vi "MGCC_comm_main.vi"() -> ()   [LabVIEW 2016]
uses:
  <vilib>/DNP3/DNP3_Master/Operation Mode.ctl
  <vilib>/DNP3/DNP3_Master/Poll Binary Input Variation.ctl
  <vilib>/DNP3/DNP3_Master/Analog Variation.ctl
  <vilib>/DNP3/DNP3_Master/Poll Analog Input Variation.ctl
  <vilib>/DNP3/DNP3_Master/Response Type.ctl
  <vilib>/DNP3/DNP3_Master/Start Stop.ctl
  <vilib>/DNP3/DNP3_Master/Analog Info.ctl
  Finite State Machine/Sub-VIs/MGCC_FntStaMach_gobal.vi
  Global communication.vi
  Global communication output.vi
  DNP3 communication files/MGCC Communication Files/DNP3_Master_Station_MGCC.lvlib
  <vilib>/DNP3/DNP3_Master.lvlib
  MGCC_Global_communication_inputsettings .vi
  <vilib>/ErrorRing/Error Ring.xnode
  <vilib>/Utility/error.llb/Error Cluster From Error Code.vi
panel:
  in  "BESS2 P":dbl
  in  "Gen P":dbl
  in  "BESS1 P":dbl
  in  "PV P":dbl
  in  "Other":bool[](array[boolean])=[FALSE, FALSE, FALSE, FALSE, FALSE, TRUE]
  out "element 2":dbl format="%#_13g"
  out "element":dbl format="%#_15g"
  in  "Gen on off":bool
  out "millisecond timer value":u32
  in  "BESS2 on off":bool
  out "Analog command":T1[][](array[typedef])=[[{"index"=0, "value"=0.0}, {"index"=1, "value"=0.0}, {"index"=2, "value"=0.0}, {"index"=3, "value"=0.0}, {"index"=4, "value"=0.0}, {"index"=5, "value"=0.0}, {"index"=6, "value"=0.0}, {"index"=7, "value"=0.0}, {"index"=0, "value"=0.0}, {"index"=0, "value"=0.0}, {"index"=0, "value"=0.0}, {"index"=0, "value"=0.0}, {"index"=0, "value"=0.0}, {"index"=0, "value"=0.0}, {"index"=0, "value"=0.0}, {"index"=0, "value"=0.0}, {"index"=0, "value"=0.0}, {"index"=0, "value"=0.0}, {"index"=0, "value"=0.0}, {"index"=0, "value"=0.0}, {"index"=0, "value"=0.0}, {"index"=0, "value"=0.0}, {"index"=0, "value"=0.0}, {"index"=0, "value"=0.0}, {"index"=0, "value"=0.0}, {"index"=0, "value"=0.0}, {"index"=0, "value"=0.0}, {"index"=0, "value"=0.0}, {"index"=0, "value"=0.0}, {"index"=0, "value"=0.0}], [{"index"=0, "value"=1.0}, {"index"=1, "value"=0.0}, {"index"=2, "value"=0.0}, {"index"=3, "value"=0.0}, {"index"=4, "value"=0.0}, {"index"=5, "value"=0.0}, {"index"=6, "value"=0.0}, {"index"=7, "value"=0.0}, {"index"=8, "value"=0.0}, {"index"=9, "value"=0.0}, {"index"=10, "value"=1.0}, {"index"=11, "value"=0.0}, {"index"=12, "value"=0.0}, {"index"=13, "value"=0.0}, {"index"=14, "value"=0.0}, {"index"=15, "value"=0.0}, {"index"=16, "value"=0.0}, {"index"=17, "value"=0.0}, {"index"=18, "value"=0.0}, {"index"=19, "value"=0.0}, {"index"=20, "value"=0.0}, {"index"=21, "value"=0.0}, {"index"=22, "value"=0.0}, {"index"=23, "value"=0.0}, {"index"=24, "value"=0.0}, {"index"=25, "value"=0.0}, {"index"=26, "value"=0.0}, {"index"=27, "value"=0.0}, {"index"=28, "value"=0.0}, {"index"=29, "value"=0.0}], [{"index"=0, "value"=1.0}, {"index"=1, "value"=0.0}, {"index"=2, "value"=0.0}, {"index"=3, "value"=0.0}, {"index"=4, "value"=0.0}, {"index"=5, "value"=0.0}, {"index"=6, "value"=0.0}, {"index"=7, "value"=0.0}, {"index"=8, "value"=0.0}, {"index"=9, "value"=0.0}, {"index"=0, "value"=0.0}, {"index"=0, "value"=0.0}, {"index"=0, "value"=0.0}, {"index"=0, "value"=0.0}, {"index"=0, "value"=0.0}, {"index"=0, "value"=0.0}, {"index"=0, "value"=0.0}, {"index"=0, "value"=0.0}, {"index"=0, "value"=0.0}, {"index"=0, "value"=0.0}, {"index"=0, "value"=0.0}, {"index"=0, "value"=0.0}, {"index"=0, "value"=0.0}, {"index"=0, "value"=0.0}, {"index"=0, "value"=0.0}, {"index"=0, "value"=0.0}, {"index"=0, "value"=0.0}, {"index"=0, "value"=0.0}, {"index"=0, "value"=0.0}, {"index"=0, "value"=0.0}]] {"value" format="%#_15f"}
  out "Analog Input 3":dbl[](array[numeric])=[0.0, 0.9942618583829594, 1.0001042537592353, 1.0057560606347744, 0.000339122595439996, 0.0004791410400245842, 0.0008348392532100933, 59.99916524340338, 59.947156617325426, 2.717283070965033, 0.00015278200018709444, -7.123436925011697e-08, 0.0, 0.0, 0.0, 0.0, 0.00033913312014400264, 0.0004791153238902122, 0.0008348307722615329, 4.282069400587955e-07, 4.985840358304346e-07, 1.0429850076204365e-06, 59.94715659629209, 59.94905915422042, -0.15889133301638747, 7.411408048091064e-11, 7.148414556889509e-15, 0.0, 0.0, 0.0, 0.0, 0.00033956781057346825, 0.0004788659040752981, 0.000835003196198178, 1.063294798850192, 0.9804226659808449, 1.0659806618953438, 59.94719306165103, 59.98302369947874, -0.2159221057021128, -8.429146107164405e-08, -1.427083545010438e-08, 0.0, 0.0, 0.0, 0.0, 0.00033909459301970524, 0.0004791936139860199, 0.0008348631578916183, 5.653331029079946e-07, 6.600727141525967e-07, 1.357194267764842e-06, 59.94715897696543, 59.94891873278328, -0.18916293881394353, 7.409342773801824e-11, 1.1504407229014506e-14, 0.0, 0.0, 0.0, 0.0, 0.000339095734403488, 0.0004791957386209789, 0.0008348655488295841, 1.839569633862611e-07, 2.1493942739428542e-07, 4.422781944829691e-07, 59.94715896582638, 59.948980263380776, -0.2257567623665988, 7.41726158569388e-11, 4.555747121595991e-15, 0.0, 0.0, 0.0, 0.0, 1.8399165630995902e-07, 2.1478488850041284e-07, 4.4219588987092504e-07, 6.415774786434966e-11, 6.120015633183977e-11, 1.5017272102437864e-10, 59.948980178541134, 59.95073734635259, -0.13958050074379713, 1.9844258378868394e-17, 4.494075267469924e-22, 0.0, 0.0, 0.0, 0.0, 0.00033884739110626985, 0.00047973946656970325, 0.000835116655298238, 4.794540398320527e-06, 1.6946200635754802, 1.72911748501882, 59.947176698087354, 59.963130270567625, 0.782636575168802, -1.1743140350345762e-07, -6.601684719983745e-08, 0.0, 0.0, 0.0, 0.0, 0.0, 0.0, 0.0, 0.0, 0.0, 0.0, 0.0, 0.0, 0.0, 0.0, 0.0, 0.0, 0.0, 0.0]
  in  "LC1_MS_Network_Settings 3":T2={"Outstation IP"="160.36.56.200", "DNP3 Port"=18000, "DNP3 Master Address"=3, "DNP3 Outstation Address"=1}
  in  "LC1_MS_DNP3_Settings 3":T7={"Binary Out Mode"=6, "Binary In Variation"=0, "Analog Out Variation"=4, "Analog Out Mode"=6, "Analog In Variation"=6} {"Analog In Variation" items=["Default", "32-bit with Flag", "16-bit with Flag", "32-bit without Flag", "16-bit without Flag", "Single-prec with Flag", "Double-prec with Flag"]; "Analog Out Mode" items=["SBO"=0, "Select"=3, "Operate"=4, "Direct"=5, "Direct No Ack"=6]; "Analog Out Variation" items=["32-bit"=1, "16-bit"=2, "Single-prec"=3, "Double-prec"=4]; "Binary In Variation" items=["Default", "Packed Format", "With Flags"]; "Binary Out Mode" items=["SBO"=0, "Select"=3, "Operate"=4, "Direct"=5, "Direct No Ack"=6]}
  in  "ENABLE MS 3":bool=TRUE
  out "LC1_MS_TX_Status_Binary 3":T8=enum."Cancel"
  out "LC1_MS_TX_Status_Analog 3":T8=enum."Success"
  out "LC1_MS_RX_Status_Binary 3":T8=enum."Cancel"
  out "LC1_MS_RX_Status_Analog 3":T8=enum."Success"
  in  "Poll Enable 3":T9={"En_Rx_An"=TRUE, "En_Tx_An"=TRUE, "En_Rx_Di"=FALSE, "En_Tx_Di"=FALSE}
  in  "RESET MS 3":bool caption="Reset Outstation"
  out "Array":T11(array[cluster])=[{"DNP3 channel"="Master/Channel 160.36.56.200: 18000", "DNP3 master"="Master", "DNP3 master session"="Master/Channel 160.36.56.200: 18000/Master Session 3-1", "DNP3 command"="Master/Channel 160.36.56.200: 18000/Master Session 3-1/Command ", "MS_Network_Settings_Initial"={"Outstation IP"="160.36.56.200", "DNP3 Port"=18000, "DNP3 Master Address"=3, "DNP3 Outstation Address"=1}, "Ping status"=enum."Success", "PollD"=[{"start"=0, "stop"=0}], "PollA"=[{"start"=0, "stop"=119}], "error out"={"status"=FALSE, "code"=5103, "source"="DNP3_Master_Station_MGCC.lvlib:LC1_MS_Main.vi:580001<ERR>\nCommunication timeout\n\n\n<b>Complete call chain:</b>\n     DNP3_Master_Station_MGCC.lvlib:LC1_MS_Main.vi:580001\n     MGCC_comm_main.vi"}, "MS_RESET_IND"=FALSE}, {"DNP3 channel"="Master #1/Channel 160.36.58.216: 18000", "DNP3 master"="Master #1", "DNP3 master session"="Master #1/Channel 160.36.58.216: 18000/Master Session 12345-54321", "DNP3 command"="Master #1/Channel 160.36.58.216: 18000/Master Session 12345-54321/Command ", "MS_Network_Settings_Initial"={"Outstation IP"="160.36.58.216", "DNP3 Port"=18000, "DNP3 Master Address"=12345, "DNP3 Outstation Address"=54321}, "Ping status"=enum."Success", "PollD"=[{"start"=0, "stop"=0}], "PollA"=[{"start"=0, "stop"=0}, {"start"=0, "stop"=0}, {"start"=0, "stop"=0}, {"start"=0, "stop"=0}, {"start"=0, "stop"=0}, {"start"=0, "stop"=0}, {"start"=0, "stop"=0}, {"start"=0, "stop"=0}, {"start"=0, "stop"=0}, {"start"=0, "stop"=0}, {"start"=0, "stop"=0}, {"start"=0, "stop"=0}, {"start"=0, "stop"=0}, {"start"=0, "stop"=0}, {"start"=0, "stop"=0}, {"start"=0, "stop"=0}, {"start"=0, "stop"=0}, {"start"=0, "stop"=0}, {"start"=0, "stop"=0}, {"start"=0, "stop"=0}, {"start"=0, "stop"=0}, {"start"=0, "stop"=0}, {"start"=0, "stop"=0}, {"start"=0, "stop"=0}, {"start"=0, "stop"=0}, {"start"=0, "stop"=0}, {"start"=0, "stop"=0}, {"start"=0, "stop"=0}, {"start"=0, "stop"=0}, {"start"=0, "stop"=0}, {"start"=0, "stop"=0}, {"start"=0, "stop"=0}, {"start"=0, "stop"=0}, {"start"=0, "stop"=0}, {"start"=0, "stop"=0}, {"start"=0, "stop"=0}, {"start"=0, "stop"=0}, {"start"=0, "stop"=0}, {"start"=0, "stop"=0}, {"start"=0, "stop"=0}, {"start"=0, "stop"=0}, {"start"=0, "stop"=0}, {"start"=0, "stop"=0}, {"start"=0, "stop"=0}, {"start"=0, "stop"=0}, {"start"=0, "stop"=0}, {"start"=0, "stop"=0}, {"start"=0, "stop"=0}, {"start"=0, "stop"=0}, {"start"=0, "stop"=0}, {"start"=0, "stop"=0}, {"start"=0, "stop"=0}, {"start"=0, "stop"=0}, {"start"=0, "stop"=0}, {"start"=0, "stop"=0}, {"start"=0, "stop"=0}, {"start"=0, "stop"=0}, {"start"=0, "stop"=0}, {"start"=0, "stop"=0}, {"start"=0, "stop"=0}, {"start"=0, "stop"=0}, {"start"=0, "stop"=0}, {"start"=0, "stop"=0}, {"start"=0, "stop"=0}, {"start"=0, "stop"=0}, {"start"=0, "stop"=0}, {"start"=0, "stop"=0}, {"start"=0, "stop"=0}, {"start"=0, "stop"=0}, {"start"=0, "stop"=0}, {"start"=0, "stop"=0}, {"start"=0, "stop"=0}, {"start"=0, "stop"=0}, {"start"=0, "stop"=0}, {"start"=0, "stop"=0}, {"start"=0, "stop"=0}, {"start"=0, "stop"=0}, {"start"=0, "stop"=0}, {"start"=0, "stop"=0}, {"start"=0, "stop"=0}, {"start"=0, "stop"=0}, {"start"=0, "stop"=0}, {"start"=0, "stop"=0}, {"start"=0, "stop"=0}, {"start"=0, "stop"=0}, {"start"=0, "stop"=0}, {"start"=0, "stop"=0}, {"start"=0, "stop"=0}, {"start"=0, "stop"=0}, {"start"=0, "stop"=0}, {"start"=0, "stop"=0}, {"start"=0, "stop"=0}, {"start"=0, "stop"=0}, {"start"=0, "stop"=0}, {"start"=0, "stop"=0}, {"start"=0, "stop"=0}, {"start"=0, "stop"=0}, {"start"=0, "stop"=0}, {"start"=0, "stop"=0}, {"start"=0, "stop"=0}, {"start"=0, "stop"=19}], "error out"={"status"=FALSE, "code"=0, "source"=""}, "MS_RESET_IND"=FALSE}, {"DNP3 channel"="Master #2/Channel 160.36.58.123: 18000", "DNP3 master"="Master #2", "DNP3 master session"="Master #2/Channel 160.36.58.123: 18000/Master Session 12340-54320", "DNP3 command"="Master #2/Channel 160.36.58.123: 18000/Master Session 12340-54320/Command ", "MS_Network_Settings_Initial"={"Outstation IP"="160.36.58.123", "DNP3 Port"=18000, "DNP3 Master Address"=12340, "DNP3 Outstation Address"=54320}, "Ping status"=enum."Success", "PollD"=[{"start"=0, "stop"=0}], "PollA"=[{"start"=0, "stop"=0}, {"start"=0, "stop"=0}, {"start"=0, "stop"=0}, {"start"=0, "stop"=0}, {"start"=0, "stop"=0}, {"start"=0, "stop"=0}, {"start"=0, "stop"=0}, {"start"=0, "stop"=0}, {"start"=0, "stop"=0}, {"start"=0, "stop"=0}, {"start"=0, "stop"=0}, {"start"=0, "stop"=0}, {"start"=0, "stop"=0}, {"start"=0, "stop"=0}, {"start"=0, "stop"=0}, {"start"=0, "stop"=0}, {"start"=0, "stop"=0}, {"start"=0, "stop"=0}, {"start"=0, "stop"=0}, {"start"=0, "stop"=0}, {"start"=0, "stop"=0}, {"start"=0, "stop"=0}, {"start"=0, "stop"=0}, {"start"=0, "stop"=0}, {"start"=0, "stop"=0}, {"start"=0, "stop"=0}, {"start"=0, "stop"=0}, {"start"=0, "stop"=0}, {"start"=0, "stop"=0}, {"start"=0, "stop"=0}, {"start"=0, "stop"=0}, {"start"=0, "stop"=0}, {"start"=0, "stop"=0}, {"start"=0, "stop"=0}, {"start"=0, "stop"=0}, {"start"=0, "stop"=0}, {"start"=0, "stop"=0}, {"start"=0, "stop"=0}, {"start"=0, "stop"=0}, {"start"=0, "stop"=0}, {"start"=0, "stop"=0}, {"start"=0, "stop"=0}, {"start"=0, "stop"=0}, {"start"=0, "stop"=0}, {"start"=0, "stop"=0}, {"start"=0, "stop"=0}, {"start"=0, "stop"=0}, {"start"=0, "stop"=0}, {"start"=0, "stop"=0}, {"start"=0, "stop"=0}, {"start"=0, "stop"=0}, {"start"=0, "stop"=0}, {"start"=0, "stop"=0}, {"start"=0, "stop"=0}, {"start"=0, "stop"=0}, {"start"=0, "stop"=0}, {"start"=0, "stop"=0}, {"start"=0, "stop"=0}, {"start"=0, "stop"=0}, {"start"=0, "stop"=0}, {"start"=0, "stop"=0}, {"start"=0, "stop"=0}, {"start"=0, "stop"=0}, {"start"=0, "stop"=0}, {"start"=0, "stop"=0}, {"start"=0, "stop"=0}, {"start"=0, "stop"=0}, {"start"=0, "stop"=0}, {"start"=0, "stop"=0}, {"start"=0, "stop"=0}, {"start"=0, "stop"=0}, {"start"=0, "stop"=0}, {"start"=0, "stop"=0}, {"start"=0, "stop"=0}, {"start"=0, "stop"=0}, {"start"=0, "stop"=0}, {"start"=0, "stop"=0}, {"start"=0, "stop"=0}, {"start"=0, "stop"=0}, {"start"=0, "stop"=0}, {"start"=0, "stop"=0}, {"start"=0, "stop"=0}, {"start"=0, "stop"=0}, {"start"=0, "stop"=0}, {"start"=0, "stop"=0}, {"start"=0, "stop"=0}, {"start"=0, "stop"=0}, {"start"=0, "stop"=0}, {"start"=0, "stop"=0}, {"start"=0, "stop"=0}, {"start"=0, "stop"=0}, {"start"=0, "stop"=0}, {"start"=0, "stop"=0}, {"start"=0, "stop"=0}, {"start"=0, "stop"=0}, {"start"=0, "stop"=0}, {"start"=0, "stop"=0}, {"start"=0, "stop"=0}, {"start"=0, "stop"=0}, {"start"=0, "stop"=0}, {"start"=0, "stop"=0}, {"start"=0, "stop"=0}, {"start"=0, "stop"=0}, {"start"=0, "stop"=0}, {"start"=0, "stop"=0}, {"start"=0, "stop"=0}, {"start"=0, "stop"=0}, {"start"=0, "stop"=0}, {"start"=0, "stop"=0}, {"start"=0, "stop"=0}, {"start"=0, "stop"=0}, {"start"=0, "stop"=0}, {"start"=0, "stop"=0}, {"start"=0, "stop"=0}, {"start"=0, "stop"=5}], "error out"={"status"=FALSE, "code"=0, "source"=""}, "MS_RESET_IND"=FALSE}]
  out "Active Station":i32=2
  out "error out 3":errorcluster
  out "error out 2":errorcluster
  out "error out":errorcluster
  out "Analog Input 2":dbl[](array[numeric])=[0.0, 1.0369912716646734, 77.34322814800805, 0.0, 0.0, 0.5, 0.0, 0.0, 0.0, 0.0, 0.0, 0.0, 0.0, 0.0, 0.0, 0.0, 0.0, 0.0, 0.0, 0.0, 0.0, 0.0, 0.0, 0.0, 0.0, 0.0, 0.0, 0.0, 0.0, 0.0, 0.0, 0.0, 0.0, 0.0, 0.0, 0.0, 0.0, 0.0, 0.0, 0.0, 0.0, 0.0, 0.0, 0.0, 0.0, 0.0, 0.0, 0.0, 0.0, 0.0, 0.0, 0.0, 0.0, 0.0, 0.0, 0.0, 0.0, 0.0, 0.0, 0.0, 0.0, 0.0, 0.0, 0.0, 0.0, 0.0, 0.0, 0.0, 0.0, 0.0, 0.0, 0.0, 0.0, 0.0, 0.0, 0.0, 0.0, 0.0, 0.0, 0.0, 0.0, 0.0, 0.0, 0.0, 0.0, 0.0, 0.0, 0.0, 0.0, 0.0, 0.0, 0.0, 0.0, 0.0, 0.0, 0.0, 0.0, 0.0, 0.0, 0.0, 0.0, 0.0, 0.0, 0.0, 0.0, 0.0, 0.0, 0.0, 0.0, 0.0, 0.0, 0.0, 0.0, 0.0, 0.0, 0.0, 0.0, 0.0, 0.0, 0.0]
  out "Analog Input":ext[](array[numeric])=[1.0, 0.9417947239708155, 89.67650077398866, -10.0, -1.8175943235401064, 0.5, 0.0, 1.080207045422867, 59.972853370476514, -4.389788955450058e-06, 5.513196811079979e-06, 0.0, 0.0, 0.0, 0.0, 0.0, 0.0, 0.0, 0.0, 0.0, 1.0, 1.0, 1.0, 1.0, 1.0, 1.0, 1.0, 1.0, 1.0, 1.0, 1.0, 1.0, 1.0, 1.0, 1.0, 1.0, 1.0, 1.0, 1.0, 1.0, 1.0, 1.0, 1.0, 1.0, 1.0, 1.0, 1.0, 1.0, 1.0, 1.0, 1.0, 1.0, 1.0, 1.0, 1.0, 1.0, 1.0, 1.0, 1.0, 1.0, 1.0, 1.0, 1.0, 1.0, 1.0, 1.0, 1.0, 1.0, 1.0, 1.0, 1.0, 1.0, 1.0, 1.0, 1.0, 1.0, 1.0, 1.0, 1.0, 1.0, 1.0, 1.0, 1.0, 1.0, 1.0, 1.0, 1.0, 1.0, 1.0, 1.0, 1.0, 1.0, 1.0, 1.0, 1.0, 1.0, 1.0, 1.0, 1.0, 1.0, 1.0, 1.0, 1.0, 1.0, 1.0, 1.0, 1.0, 1.0, 1.0, 1.0, 1.0, 1.0, 1.0, 1.0, 1.0, 1.0, 1.0, 1.0, 1.0, 1.0]
  in  "LC1_MS_Network_Settings 2":T2={"Outstation IP"="10.38.59.112", "DNP3 Port"=18000, "DNP3 Master Address"=12340, "DNP3 Outstation Address"=54320}
  in  "LC1_MS_DNP3_Settings 2":T7={"Binary Out Mode"=6, "Binary In Variation"=0, "Analog Out Variation"=4, "Analog Out Mode"=6, "Analog In Variation"=6} {"Analog In Variation" items=["Default", "32-bit with Flag", "16-bit with Flag", "32-bit without Flag", "16-bit without Flag", "Single-prec with Flag", "Double-prec with Flag"]; "Analog Out Mode" items=["SBO"=0, "Select"=3, "Operate"=4, "Direct"=5, "Direct No Ack"=6]; "Analog Out Variation" items=["32-bit"=1, "16-bit"=2, "Single-prec"=3, "Double-prec"=4]; "Binary In Variation" items=["Default", "Packed Format", "With Flags"]; "Binary Out Mode" items=["SBO"=0, "Select"=3, "Operate"=4, "Direct"=5, "Direct No Ack"=6]}
  in  "ENABLE MS 2":bool=TRUE
  out "MS SETTINGS CHANGED 2":bool
  out "LC1_MS_TX_Status_Binary 2":T8=enum."Cancel"
  out "LC1_MS_TX_Status_Analog 2":T8=enum."Success"
  out "LC1_MS_RX_Status_Binary 2":T8=enum."Cancel"
  out "LC1_MS_RX_Status_Analog 2":T8=enum."Success"
  out "RESET MS IND 2":bool
  in  "Poll Enable 2":T9={"En_Rx_An"=TRUE, "En_Tx_An"=TRUE, "En_Rx_Di"=FALSE, "En_Tx_Di"=FALSE}
  in  "RESET MS 2":bool caption="Reset Outstation"
  in  "Poll Enable":T9={"En_Rx_An"=TRUE, "En_Tx_An"=TRUE, "En_Rx_Di"=FALSE, "En_Tx_Di"=FALSE}
  out "Numeric":i32=132
  out "RESET MS IND":bool
  out "LC1_MS_RX_Status_Analog":T8=enum."Success"
  out "LC1_MS_RX_Status_Binary":T8=enum."Cancel"
  out "LC1_MS_TX_Status_Analog":T8=enum."Success"
  out "LC1_MS_TX_Status_Binary":T8=enum."Cancel"
  out "MS SETTINGS CHANGED":bool
  in  "RESET MS":bool caption="Reset Outstation"
  in  "ENABLE MS":bool=TRUE
  in  "LC1_MS_DNP3_Settings":T7={"Binary Out Mode"=6, "Binary In Variation"=0, "Analog Out Variation"=4, "Analog Out Mode"=6, "Analog In Variation"=6} {"Analog In Variation" items=["Default", "32-bit with Flag", "16-bit with Flag", "32-bit without Flag", "16-bit without Flag", "Single-prec with Flag", "Double-prec with Flag"]; "Analog Out Mode" items=["SBO"=0, "Select"=3, "Operate"=4, "Direct"=5, "Direct No Ack"=6]; "Analog Out Variation" items=["32-bit"=1, "16-bit"=2, "Single-prec"=3, "Double-prec"=4]; "Binary In Variation" items=["Default", "Packed Format", "With Flags"]; "Binary Out Mode" items=["SBO"=0, "Select"=3, "Operate"=4, "Direct"=5, "Direct No Ack"=6]}
  in  "LC1_MS_Network_Settings":T2={"Outstation IP"="10.38.59.111", "DNP3 Port"=18000, "DNP3 Master Address"=12345, "DNP3 Outstation Address"=54321}
  in  "Manually control Relays":bool
  in  "PV on off":bool
  in  "Manually control sources":bool
  in  "BESS1 on off":bool
  in  "Relay":bool[](array[boolean])=[FALSE, FALSE, FALSE, FALSE, FALSE, FALSE, FALSE, FALSE, FALSE, FALSE]
  # "Copyright <2020> <The University of Tennessee at Knoxville and the University of Tennessee Research Foundation>\n\nRedistribution and use in source and binary forms, with or without modification, are permitted provided that the following conditions are met:\n\n1. Redistributions of source code must retain the above copyright notice, this list of conditions and the following disclaimer.\n\n2. Redistributions in binary form must reproduce the above copyright notice, this list of conditions and the following disclaimer in the documentation and/or other materials provided with the distribution.\n\n3. Neither the name of the copyright holder nor the names of its contributors may be used to endorse or promote products derived from this software without specific prior written permission.\n\nTHIS SOFTWARE IS PROVIDED BY THE COPYRIGHT HOLDERS AND CONTRIBUTORS \"AS IS\" AND ANY EXPRESS OR IMPLIED WARRANTIES, INCLUDING, BUT NOT LIMITED TO, THE IMPLIED WARRANTIES OF MERCHANTABILITY AND FITNESS FOR A PARTICULAR PURPOSE ARE DISCLAIMED. IN NO EVENT SHALL THE COPYRIGHT HOLDER OR CONTRIBUTORS BE LIABLE FOR ANY DIRECT, INDIRECT, INCIDENTAL, SPECIAL, EXEMPLARY, OR CONSEQUENTIAL DAMAGES (INCLUDING, BUT NOT LIMITED TO, PROCUREMENT OF SUBSTITUTE GOODS OR SERVICES; LOSS OF USE, DATA, OR PROFITS; OR BUSINESS INTERRUPTION) HOWEVER CAUSED AND ON ANY THEORY OF LIABILITY, WHETHER IN CONTRACT, STRICT LIABILITY, OR TORT (INCLUDING NEGLIGENCE OR OTHERWISE) ARISING IN ANY WAY OUT OF THE USE OF THIS SOFTWARE, EVEN IF ADVISED OF THE POSSIBILITY OF SUCH DAMAGE."
  # "LC2"
  # "LC1"
  # "IntelliRupter"
  # "Settings Changed; Reset to Update"
  # "1"
  # "fault 3 (L6)"
  # "2"
  # "fault 5 (10)"
  # "3"
  # "fault 6 (L11)"
  # "4"
  # "fault 7 (L8)"
  # "5"
  # "reset"
  # "6"
  # "grid enable"
  # "7"
  # "8"
  # "Gnd trans1"
  # "Gnd trans2"
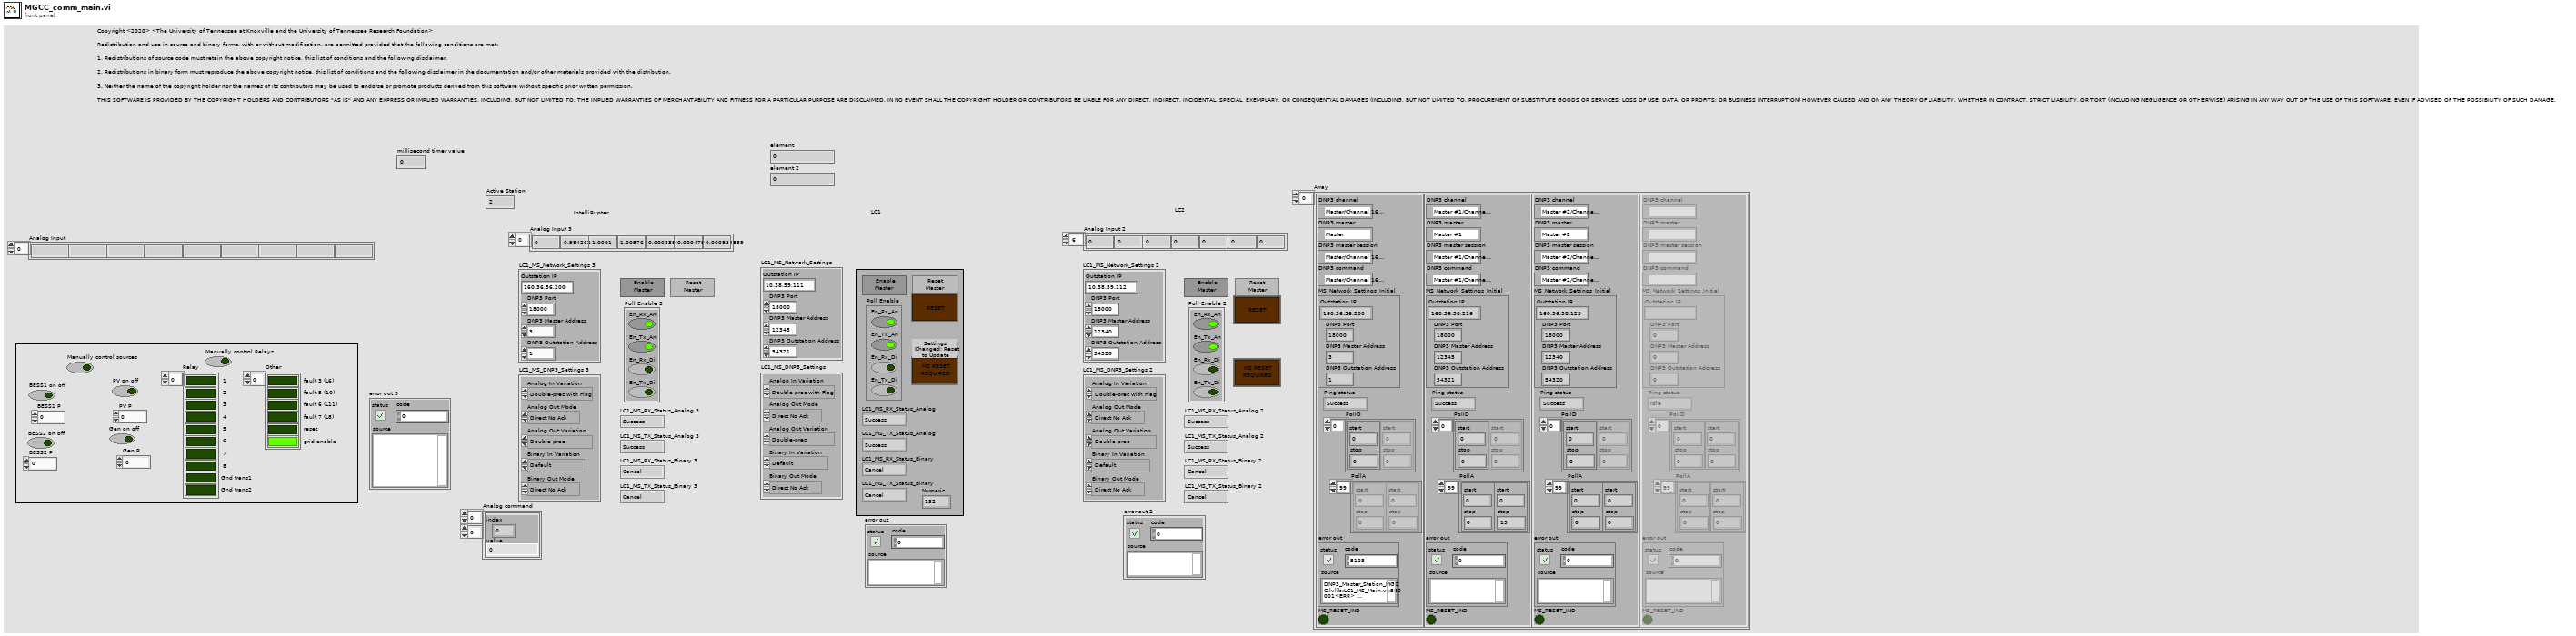
[diagram p1: front panel]
types:
  T1 = typedef "DNP3_Master.lvlib/Analog Info.ctl" = cluster{"index":u16, "value":dbl}
  T2 = cluster{"Outstation IP":string, "DNP3 Port":u16, "DNP3 Master Address":u16, "DNP3 Outstation Address":u16}
  T3 = typedef "DNP3_Master.lvlib/Operation Mode.ctl" = u8
  T4 = typedef "DNP3_Master.lvlib/Poll Binary Input Variation.ctl" = u8
  T5 = typedef "DNP3_Master.lvlib/Analog Variation.ctl" = u8
  T6 = typedef "DNP3_Master.lvlib/Poll Analog Input Variation.ctl" = u8
  T7 = cluster{"Binary Out Mode":T3, "Binary In Variation":T4, "Analog Out Variation":T5, "Analog Out Mode":T3, "Analog In Variation":T6}
  T8 = typedef "DNP3_Master.lvlib/Response Type.ctl" = enum16{"Idle", "Buffering", "Pending", "Success", "Failure", "Mismatch", "Status Code", "IIN", "Timeout", "Cancel"}
  T9 = cluster{"En_Rx_An":bool, "En_Tx_An":bool, "En_Rx_Di":bool, "En_Tx_Di":bool}
  T10 = typedef "DNP3_Master.lvlib/Start Stop.ctl" = cluster{"start":u16, "stop":u16}
  T11 = cluster{"DNP3 channel":refnum<k21>, "DNP3 master":refnum<k21>, "DNP3 master session":refnum<k21>, "DNP3 command":refnum<k21>, "MS_Network_Settings_Initial":cluster{"Outstation IP":string, "DNP3 Port":u16, "DNP3 Master Address":u16, "DNP3 Outstation Address":u16}, "Ping status":T8, "PollD":T10[], "PollA":T10[], "error out":errorcluster, "MS_RESET_IND":bool}[]
  T12 = cluster{"Binary Out Mode":T3, "Binary In Variation":T4, "Analog Out Variation":T5, "Analog Out Mode":T3, "Analog In Variation":T6}[]
  T13 = cluster{"Outstation IP":string, "DNP3 Port":u16, "DNP3 Master Address":u16, "DNP3 Outstation Address":u16}[]
  T14 = cluster{"En_Rx_An":bool, "En_Tx_An":bool, "En_Rx_Di":bool, "En_Tx_Di":bool}[]
  T15 = cluster{"response status":T8, "response status":T8, "response status":T8, "response status":T8}
  T16 = cluster{"DNP3 channel":refnum<k21>, "DNP3 master":refnum<k21>, "DNP3 master session":refnum<k21>, "DNP3 command":refnum<k21>, "MS_Network_Settings_Initial":cluster{"Outstation IP":string, "DNP3 Port":u16, "DNP3 Master Address":u16, "DNP3 Outstation Address":u16}, "Ping status":T8, "PollD":T10[], "PollA":T10[], "error out":errorcluster, "MS_RESET_IND":bool}
  T17 = cluster{string, "DNP3 port BESS":dbl, "DNP3 Master Address BESS":dbl, "DNP3 Outstation Address BESS":dbl}
  T18 = cluster{string, "DNP3 port PV":dbl, "DNP3 Master Address PV":dbl, "DNP3 Outstation Address PV":dbl}
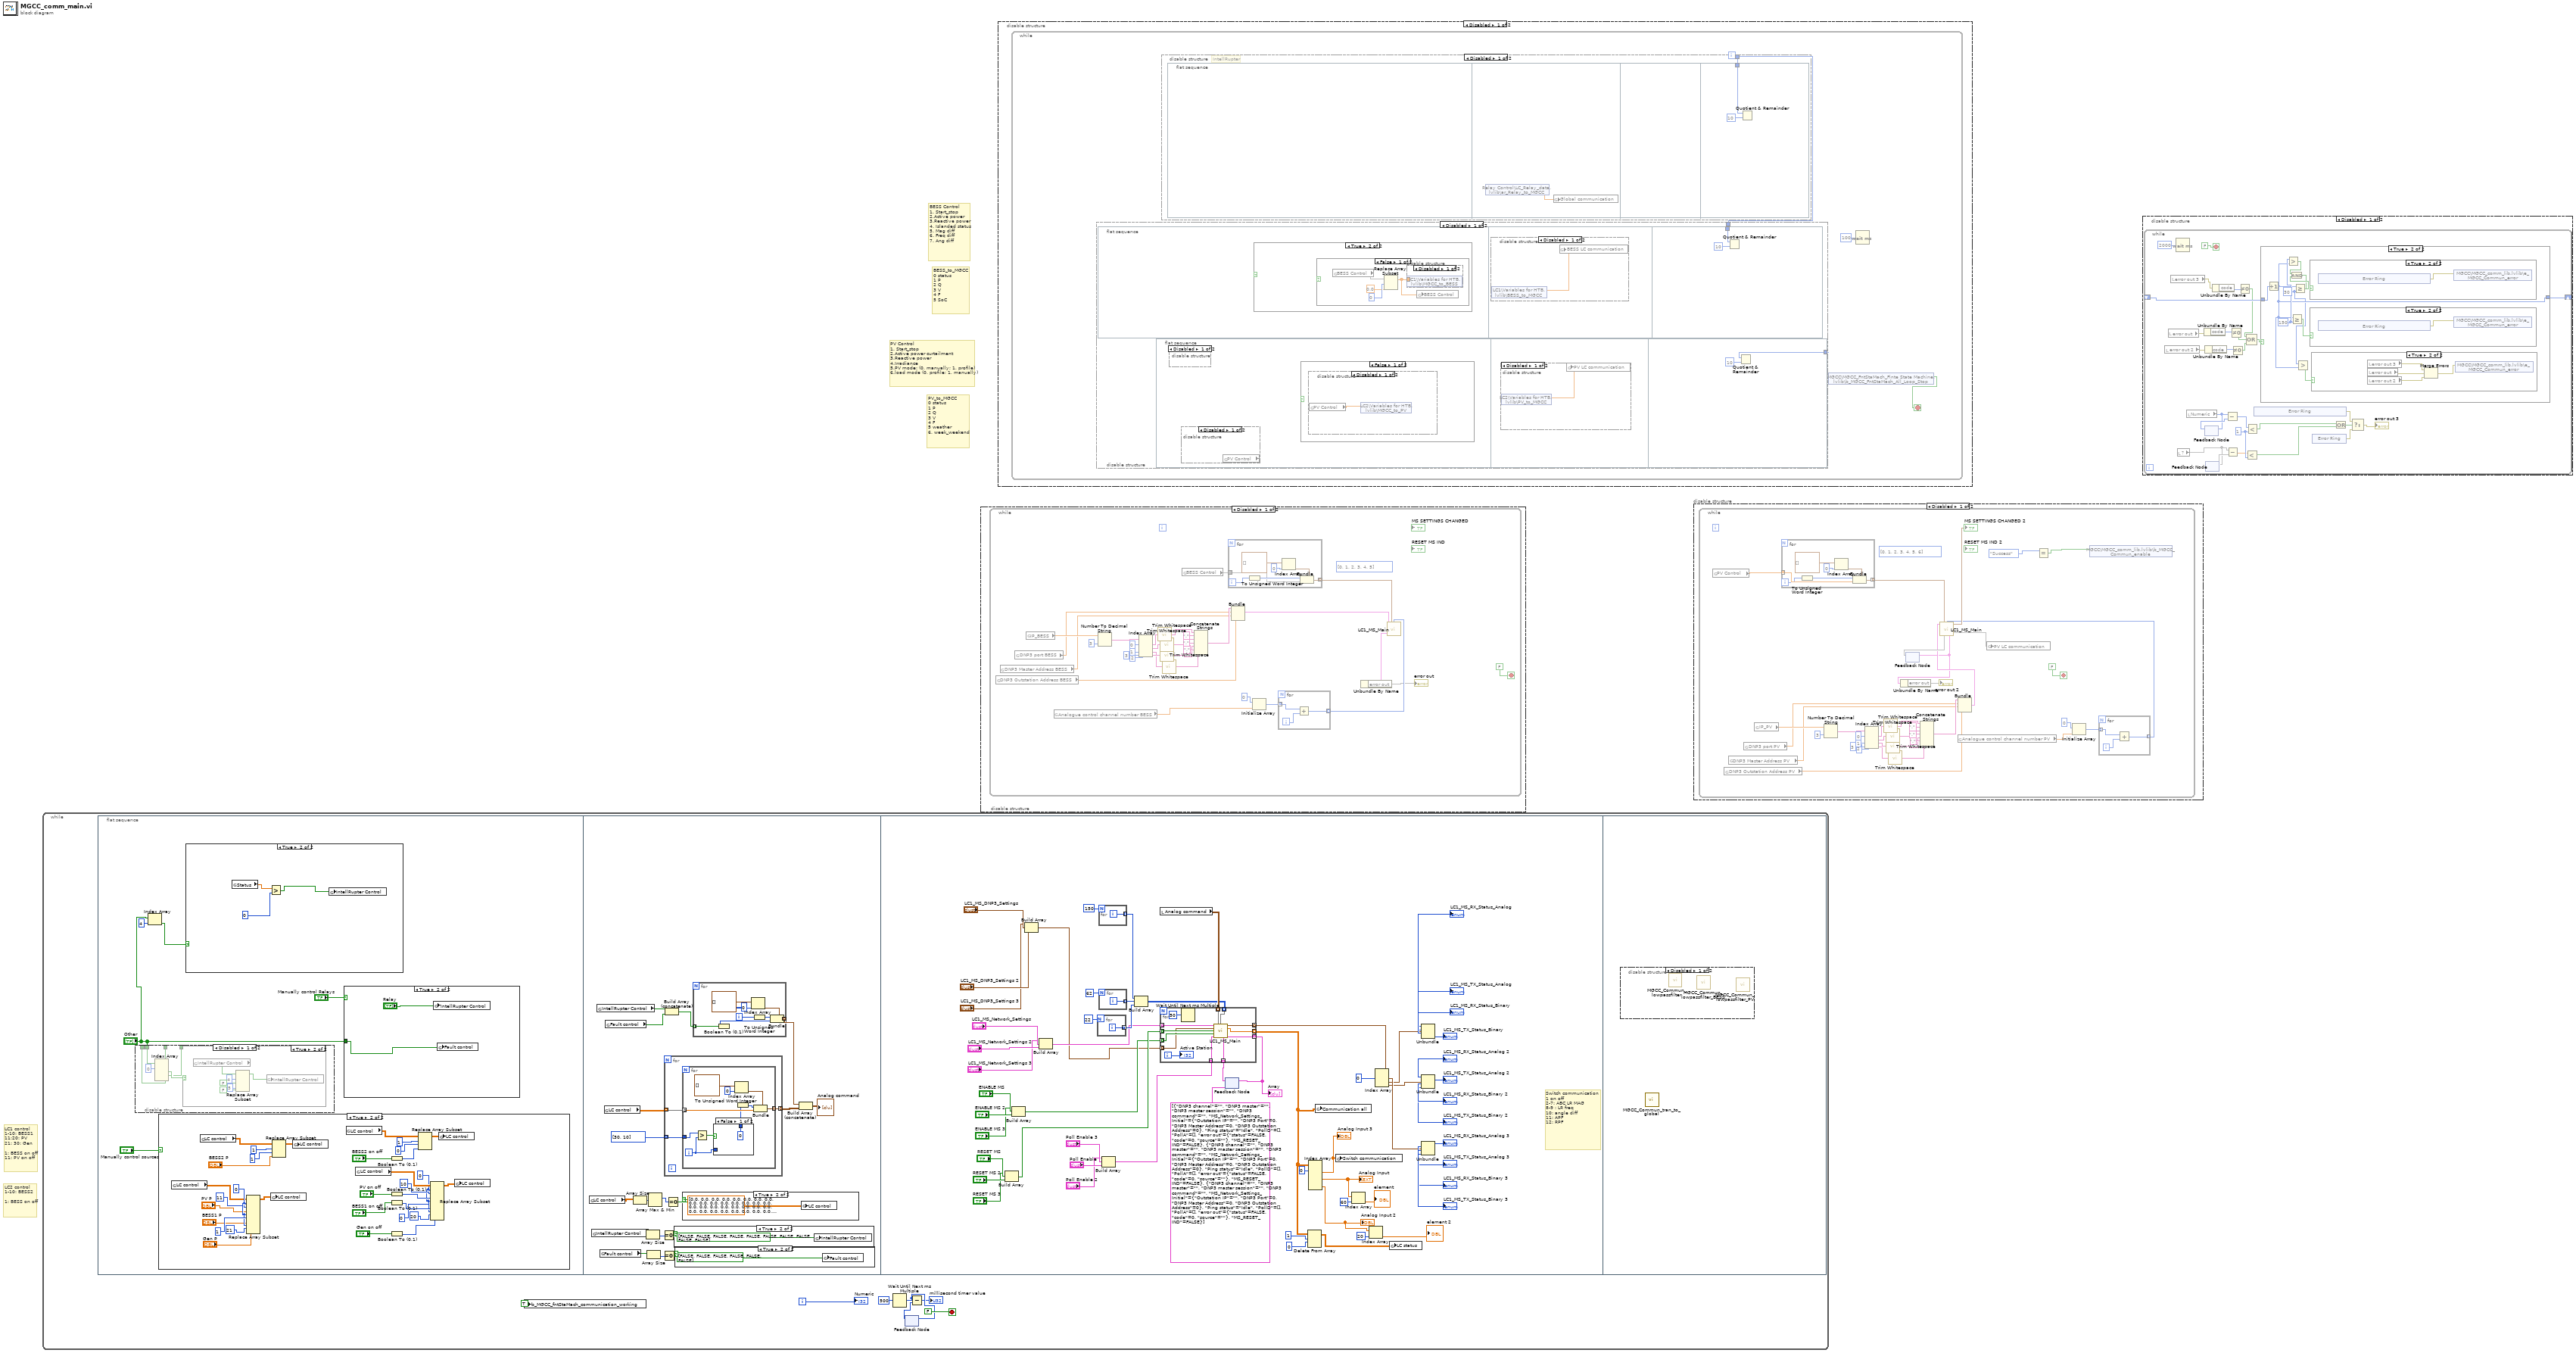
[diagram p0: block diagram]
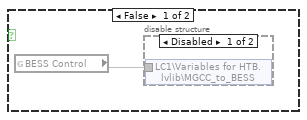
[diagram p2: hidden frame]
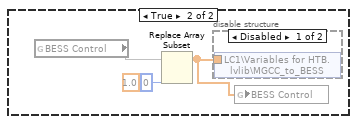
[diagram p5: hidden frame]
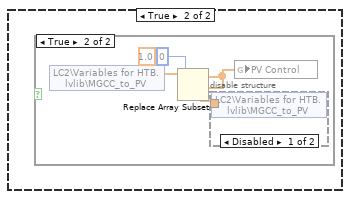
[diagram p9: hidden frame]
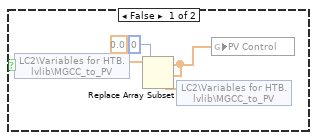
[diagram p10: hidden frame]
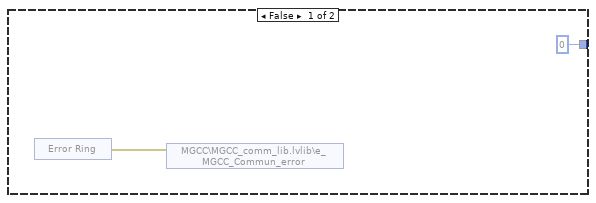
[diagram p18: hidden frame]
diagram:
  # "LC2 control\n1-10: BESS2\n\n1: BESS on off"
  # "LC1 control\n1-10: BESS1\n11:20: PV\n21: 30: Gen\n\n1: BESS on off\n11: PV on off"
  # "PV_to_MGCC\n0 status\n1 P\n2 Q\n3 V\n4 F\n5 weather\n6. week_weekend"
  # "BESS_to_MGCC\n0 status\n1 P\n2 Q\n3 V\n4 F\n5 SoC"
  # "PV Control\n1. Start_stop\n2.Active power curtailment\n3.Reactive power\n4.Irradiance\n5.PV mode: (0, manually; 1, profile)\n6.load mode (0, profile; 1, manually)"
  # "BESS Control\n1. Start_stop\n2.Active power\n3.Reactive power\n4. Islanded status\n5. Mag diff\n6. Freq diff\n7. Ang diff"
  n1 = while {
    i -> [w7]
    stop <- FALSE stop-if-true
    n2 = flat-sequence {
      frame #0 {
        n3 = disable-structure shown="Disabled" {
          disable-tunnel: "Other" -> [w20 _]
          disable-tunnel: [w18 _] -> _
          disable-tunnel: [w17 _] -> _
          disable-tunnel: [w16 _] -> _
          frame Disabled {
            n4 = Index Array(array=w20, index #1=0 ("index")) -> (element #1=w16:bool, element #2=w19:bool, element #3=w18:bool, element #4=w17:bool)  [unwired: 3 in]
            n5 = case shown="True" w19 {
              frame False {
              }
              frame True {
                n6 = global read "Global communication output.vi" "IntellRupter Control"() -> (w27:bool[])
                n7 = Replace Array Subset(array=w27, new element #1=FALSE ("new element/subarray"), index #1=4 ("index"), new element #2=FALSE ("new element/subarray"), index #2=5 ("index")) -> (w26:bool[])
                n8 = global write "Global communication output.vi" "IntellRupter Control"(w26) -> ()
              }
            }
          }
          frame Enabled {
          }
        }
        n9 = Index Array(array="Other", index=4) -> (element=w8:bool)
        n10 = case shown="True" "Manually control sources" {
          frame False {
          }
          frame True {
            w44 = 0 ("index")
            w49 = 0 ("index")
            n11 = global read "Global communication.vi" "LC control"() -> (w41:dbl[][])
            n12 = global read "Global communication.vi" "LC control"() -> (w35:dbl[][])
            n13 = Replace Array Subset(array=w41, new element #1="PV P", index (row) #1=w44, index (col) #1=11 ("index"), new element #2="BESS1 P", index (row) #2=w44, index (col) #2=1 ("index"), new element #3="Gen P", index (row) #3=w44, index (col) #3=21 ("index")) -> (w42:dbl[][])
            n14 = global write "Global communication.vi" "LC control"(w42) -> ()
            n15 = Replace Array Subset(array=w35, new element="BESS2 P", index (row)=1 ("index"), index (col)=1 ("index")) -> (w33:dbl[][])
            n16 = global write "Global communication.vi" "LC control"(w33) -> ()
            n17 = global read "Global communication.vi" "LC control"() -> (w55:dbl[][])
            n18 = global read "Global communication.vi" "LC control"() -> (w53:dbl[][])
            n19 = Boolean To (0,1)(Boolean="BESS2 on off") -> (0, 1=w59:i16)
            n20 = Boolean To (0,1)(Boolean="PV on off") -> (0, 1=w63:i16)
            n21 = Boolean To (0,1)(Boolean="BESS1 on off") -> (0, 1=w57:i16)
            n22 = Boolean To (0,1)(Boolean="Gen on off") -> (0, 1=w56:i16)
            n23 = Replace Array Subset(array=w55, new element=w59, index (row)=1 ("index"), index (col)=0 ("index")) -> (w54:dbl[][])
            n24 = Replace Array Subset(array=w53, new element #1=w63, index (row) #1=w49, index (col) #1=10 ("index"), new element #2=w57, index (row) #2=w49, index (col) #2=0 ("index"), new element #3=w56, index (row) #3=w49, index (col) #3=20 ("index")) -> (w52:dbl[][])
            n25 = global write "Global communication.vi" "LC control"(w54) -> ()
            n26 = global write "Global communication.vi" "LC control"(w52) -> ()
          }
        }
        n27 = case shown="True" w8 {
          frame False {
          }
          frame True {
            n28 = global read "Global communication.vi" "Status"() -> (w15:dbl[])
            n29 = Greater?(x=w15, y=0 ("index")) -> (0:w13:bool[])
            n30 = global write "Global communication output.vi" "IntellRupter Control"(w13) -> ()
          }
        }
        n31 = case shown="True" "Manually control Relays" {
          tunnel: "Other" -> [w28 w31]
          frame False {
            n32 = global read "Global communication output.vi" "IntellRupter Control"() -> (w29:bool[])
            n33 = disable-structure shown="Disabled" {
              frame Disabled {
                n34 = global read "Global communication output.vi" "Fault control"() -> (w30:bool[])
                n35 = local write "Other"(w30) -> ()
              }
              frame Enabled {
              }
            }
            n36 = global write "Global communication output.vi" "Fault control"(w28) -> ()
            n37 = local write "Relay"(w29) -> ()
          }
          frame True {
            n38 = global write "Global communication output.vi" "IntellRupter Control"("Relay") -> ()
            n39 = global write "Global communication output.vi" "Fault control"(w31) -> ()
          }
        }
      }
      frame #1 {
        n40 = global read "Global communication.vi" "LC control"() -> (w75:dbl[][])
        n41 = global read "Global communication output.vi" "IntellRupter Control"() -> (w78:bool[])
        n42 = global read "Global communication output.vi" "IntellRupter Control"() -> (w69:bool[])
        n43 = global read "Global communication output.vi" "Fault control"() -> (w65:bool[])
        n44 = global read "Global communication.vi" "LC control"() -> (w72:dbl[][])
        n45 = global read "Global communication output.vi" "Fault control"() -> (w68:bool[])
        n46 = Array Size(array=w75) -> (size(s)=w74:i32[])
        n47 = Array Size(array=w78) -> (size(s)=w77:i32)
        n48 = Array Size(array=w65) -> (size(s)=w66:i32)
        n49 = Array Max & Min(array=w74) -> (max index (indices)=w73:i32)  [unwired: 3 out]
        n50 = Equal To 0?(x=w77) -> (x = 0?=w76:bool)
        n51 = Equal To 0?(x=w66) -> (x = 0?=w67:bool)
        n52 = for {
          tunnel: [w86] -> w82 mode=indexing
          tunnel: w72 -> [w85] mode=indexing
          tunnel: i32[] [30, 10] ("IntellRupter Control") -> [w84] mode=indexing
          n53 = for {
            tunnel: [w96] -> w86 mode=indexing
            tunnel: w85 -> [w91] mode=indexing
            tunnel: w84 -> [w90]
            i -> [w88]
            n54 = Greater?(x=w90, y=w88) -> (0:w89:bool)
            n55 = case shown="False" w89 {
              tunnel: w88 -> [_ w98]
              tunnel: [0 w98] -> w87
              frame False {
              }
              frame True {
              }
            }
            n56 = Index Array(array=T1[] [] ("values"), index=0) -> (element=w93:T1)
            n57 = To Unsigned Word Integer(number=w87) -> (unsigned 16bit integer=w92:u16)
            n58 = Bundle(cluster=w93, "index"=w92, "value"=w91) -> (w96:T1)
          }
        }
        n59 = Build Array (concatenate)(w69, w68) -> (w70:bool[])
        n60 = Equal To 0?(x=w73) -> (x = 0?=w79:bool)
        n61 = case shown="True" w76 {
          frame False {
          }
          frame True {
            n62 = global write "Global communication output.vi" "IntellRupter Control"(bool[] [FALSE, FALSE, FALSE, FALSE, FALSE, FALSE, FALSE, FALSE, FALSE, FALSE] ("IntellRupter Control")) -> ()
          }
        }
        n63 = case shown="True" w67 {
          frame False {
          }
          frame True {
            n64 = global write "Global communication output.vi" "Fault control"(bool[] [FALSE, FALSE, FALSE, FALSE, FALSE, FALSE] ("IntellRupter Control")) -> ()
          }
        }
        n65 = case shown="True" w79 {
          frame False {
          }
          frame True {
            n66 = global write "Global communication.vi" "LC control"(dbl[][] [[0.0, 0.0, 0.0, 0.0, 0.0, 0.0, 0.0, 0.0, 0.0, 0.0, 0.0, 0.0, 0.0, 0.0, 0.0, 0.0, 0.0, 0.0, 0.0, 0.0, 0.0, 0.0, 0.0, 0.0, 0.0, 0.0, 0.0, 0.0, 0.0, 0.0, 0.0, 0.0, 0.0, 0.0, 0.0, 0.0, 0.0], [0.0, 0.0, 0.0, 0.0, 0.0, 0.0, 0.0, 0.0, 0.0, 0.0, 0.0, 0.0, 0.0, 0.0, 0.0, 0.0, 0.0, 0.0, 0.0, 0.0, 0.0, 0.0, 0.0, 0.0, 0.0, 0.0, 0.0, 0.0, 0.0, 0.0, 0.0, 0.0, 0.0, 0.0, 0.0, 0.0, 0.0]] ("LC control")) -> ()
          }
        }
        n67 = for {
          tunnel: [w108] -> w80 mode=indexing
          tunnel: w70 -> [w101] mode=indexing
          i -> [w103]
          n68 = Boolean To (0,1)(Boolean=w101) -> (0, 1=w102:i16)
          n69 = Index Array(array=T1[] [] ("values"), index=0) -> (element=w105:T1)
          n70 = To Unsigned Word Integer(number=w103) -> (unsigned 16bit integer=w104:u16)
          n71 = Bundle(cluster=w105, "index"=w104, "value"=w102) -> (w108:T1)
        }
        n72 = Build Array (concatenate)(w80, w82) -> (→"Analog command":T1[][])
      }
      frame #2 {
        # "Switch communication\n1 on off\n2-7: ABC LR MAG\n8-9 : LR freq\n10: angle diff\n11: APF\n12: RPF"
        n73 = Build Array("RESET MS 3", "RESET MS", "RESET MS 2") -> (w126:bool[])
        n74 = Build Array("ENABLE MS 3", "ENABLE MS", "ENABLE MS 2") -> (w125:bool[])
        n75 = Build Array("LC1_MS_DNP3_Settings 3", "LC1_MS_DNP3_Settings", "LC1_MS_DNP3_Settings 2") -> (w123:T12)
        n76 = Build Array("LC1_MS_Network_Settings 3", "LC1_MS_Network_Settings", "LC1_MS_Network_Settings 2") -> (w124:T13)
        n77 = for {
          N: 22 -> [_]
          tunnel: [w169] -> w148 mode=indexing
          i -> [w169]
        }
        n78 = for {
          N: 150 -> [_]
          tunnel: [w171] -> w143 mode=indexing
          i -> [w171]
        }
        n79 = for {
          N: 62 -> [_]
          tunnel: [w170] -> w146 mode=indexing
          i -> [w170]
        }
        n80 = Build Array("Poll Enable 2", "Poll Enable 3", "Poll Enable") -> (w127:T14)
        n81 = Build Array(w143, w146, w148) -> (w128:i32[][])
        n82 = local read "Analog command"() -> (w129:T1[][])
        n83 = feedback #1(T11 [{"DNP3 channel"="", "DNP3 master"="", "DNP3 master session"="", "DNP3 command"="", "MS_Network_Settings_Initial"={"Outstation IP"="", "DNP3 Port"=0, "DNP3 Master Address"=0, "DNP3 Outstation Address"=0}, "Ping status"=enum."Idle", "PollD"=[], "PollA"=[], "error out"={"status"=FALSE, "code"=0, "source"=""}, "MS_RESET_IND"=FALSE}, {"DNP3 channel"="", "DNP3 master"="", "DNP3 master session"="", "DNP3 command"="", "MS_Network_Settings_Initial"={"Outstation IP"="", "DNP3 Port"=0, "DNP3 Master Address"=0, "DNP3 Outstation Address"=0}, "Ping status"=enum."Idle", "PollD"=[], "PollA"=[], "error out"={"status"=FALSE, "code"=0, "source"=""}, "MS_RESET_IND"=FALSE}, {"DNP3 channel"="", "DNP3 master"="", "DNP3 master session"="", "DNP3 command"="", "MS_Network_Settings_Initial"={"Outstation IP"="", "DNP3 Port"=0, "DNP3 Master Address"=0, "DNP3 Outstation Address"=0}, "Ping status"=enum."Idle", "PollD"=[], "PollA"=[], "error out"={"status"=FALSE, "code"=0, "source"=""}, "MS_RESET_IND"=FALSE}]) -> (w131:T11)
        n84 = for {
          tunnel: [w184] -> w130 mode=indexing
          tunnel: w131 -> [w179] mode=indexing
          tunnel: [w181] -> w132 mode=indexing
          tunnel: [w180] -> w109 mode=indexing
          tunnel: w129 -> [w178] mode=indexing
          tunnel: w128 -> [w177] mode=indexing
          tunnel: w127 -> [w176] mode=indexing
          tunnel: w126 -> [w175] mode=indexing
          tunnel: w125 -> [w174] mode=indexing
          tunnel: w124 -> [w173] mode=indexing
          tunnel: w123 -> [w172] mode=indexing
          i -> [w183]
          n85 = Wait Until Next ms Multiple(millisecond multiple=u32 50) -> ()  [unwired: 1 out]
          n86 = call "LC1_MS_Main.vi"("MS_Network_Settings"=w173, "Analog Output"=w178, "Analog Input Indexes"=w177, "MS_DNP3_Settings"=w172, "MS_RESET"=w175, "MS_ENABLE"=w174, "Poll Enable"=w176, "DNP3 Session Feedback"=w179) -> ("Comm Status"=w181:T15, "Analog Input"=w180:dbl[], "DNP3 Session Output"=w184:T16)  [unwired: 4 in, 1 out]
          "Active Station" <- w183
        }
        "Array" <- w130
        n87 = feedback-in #1(w130) -> ()
        n88 = Delete From Array(array=w109, length=1 ("index"), index (row)=0 ("index")) -> (array with subset deleted=w116:dbl[][])  [unwired: 1 in, 1 out]
        n89 = Index Array(array=w109, index (row) #1=0 ("index")) -> (element #1=w119:dbl[], element #2=w115:dbl[], element #3=w111:dbl[])  [unwired: 5 in]
        "Analog Input" <- w115
        "Analog Input 2" <- w111
        "Analog Input 3" <- w119
        n90 = global write "Global communication.vi" "Communication all"(w109) -> ()
        n91 = global write "Global communication.vi" "Switch communication"(w119) -> ()
        n92 = Index Array(array=w115, index=60) -> (element=→"element":dbl)
        n93 = Index Array(array=w111, index=20) -> (element=→"element 2":dbl)
        n94 = Index Array(array=w132, index #1=0 ("index")) -> (element #1=w122:T15, element #2=w121:T15, element #3=w120:T15)  [unwired: 2 in]
        n95 = global write "Global communication.vi" "LC status"(w116) -> ()
        n96 = Unbundle(w121) -> ("response status"=→"LC1_MS_RX_Status_Analog":T8, "response status"=→"LC1_MS_TX_Status_Analog":T8, "response status"=→"LC1_MS_RX_Status_Binary":T8, "response status"=→"LC1_MS_TX_Status_Binary":T8)
        n97 = Unbundle(w120) -> ("response status"=→"LC1_MS_RX_Status_Analog 2":T8, "response status"=→"LC1_MS_TX_Status_Analog 2":T8, "response status"=→"LC1_MS_RX_Status_Binary 2":T8, "response status"=→"LC1_MS_TX_Status_Binary 2":T8)
        n98 = Unbundle(w122) -> ("response status"=→"LC1_MS_RX_Status_Analog 3":T8, "response status"=→"LC1_MS_TX_Status_Analog 3":T8, "response status"=→"LC1_MS_RX_Status_Binary 3":T8, "response status"=→"LC1_MS_TX_Status_Binary 3":T8)
      }
      frame #3 {
        n99 = disable-structure shown="Disabled" {
          frame Disabled {
            n100 = call "MGCC_Commun_lowpassfilter.vi"() -> ()  [unwired: 12 in]
            n101 = call "MGCC_Commun_lowpassfilter_BESS.vi"() -> ()  [unwired: 12 in]
            n102 = call "MGCC_Commun_lowpassfilter_PV.vi"() -> ()  [unwired: 12 in]
          }
          frame Enabled {
          }
        }
        n103 = call "MGCC_Commun_tran_to_global.vi"() -> ()  [unwired: 12 in]
      }
    }
    n104 = global write "MGCC_FntStaMach_gobal.vi" "b_MGCC_fntStaMach_communication_working"(TRUE ("b_MGCC_fntStaMach_ModelMgmt_done")) -> ()
    n105 = Wait Until Next ms Multiple(millisecond multiple=u32 500) -> (millisecond timer value=w3:u32)
    n106 = feedback-in #2(w3) -> ()
    n107 = feedback #2() -> (w4:u32)  [unwired: 1 in]
    n108 = Subtract(x=w3, y=w4) -> (x-y=→"millisecond timer value":u32)
    "Numeric" <- w7
  }
  n109 = disable-structure shown="Disabled" {
    frame Disabled {
      n110 = while {
        i -> [w223]
        stop <- FALSE stop-if-true
        (unwired) u16[] [0, 1, 2, 3, 4, 5] ("Analog Input Indexes")
        n111 = global read "MGCC_Global_communication_inputsettings .vi" "DNP3 Outstation Address BESS"() -> (w193:dbl)
        n112 = global read "MGCC_Global_communication_inputsettings .vi" "DNP3 Master Address BESS"() -> (w194:dbl)
        n113 = global read "MGCC_Global_communication_inputsettings .vi" "DNP3 port BESS"() -> (w195:dbl)
        n114 = global read "MGCC_Global_communication_inputsettings .vi" "IP_BESS"() -> (w197:dbl[])
        n115 = global read "MGCC_Global_communication_inputsettings .vi" "Analogue control channel number BESS"() -> (w189:dbl)
        n116 = Number To Decimal String(number=w197, width (-)=i16 3) -> (decimal integer string=w214:string[])
        n117 = Index Array(array=w214, index #1=0 ("index"), index #2=1 ("index"), index #3=2 ("index"), index #4=3 ("index")) -> (element #1=w206:string, element #2=w204:string, element #3=w202:string, element #4=w200:string)
        n118 = call <vilib>:"Trim Whitespace.vi"("string"=w206) -> ("trimmed string"=w205:string)  [unwired: 1 in]
        n119 = call <vilib>:"Trim Whitespace.vi"("string"=w204) -> ("trimmed string"=w203:string)  [unwired: 1 in]
        n120 = call <vilib>:"Trim Whitespace.vi"("string"=w202) -> ("trimmed string"=w201:string)  [unwired: 1 in]
        n121 = call <vilib>:"Trim Whitespace.vi"("string"=w200) -> ("trimmed string"=w199:string)  [unwired: 1 in]
        n122 = global read "Global communication output.vi" "BESS Control"() -> (w216)
        n123 = Concatenate Strings(w205, "." ("string"), w203, "." ("string"), w201, "." ("string"), w199) -> (w196:string)
        n124 = for {
          tunnel: [w234] -> w215 mode=indexing
          tunnel: w216 -> [w229]
          i -> [w228]
          n125 = To Unsigned Word Integer(number=w228) -> (unsigned 16bit integer=w230:u16)
          n126 = Index Array(array=T1[] [] ("values"), index=0) -> (element=w231:T1)
          n127 = Bundle(cluster=w231, "index"=w230, "value"=w229) -> (w234:T1)
        }
        n128 = Bundle(w196, "DNP3 port BESS"=w195, "DNP3 Master Address BESS"=w194, "DNP3 Outstation Address BESS"=w193) -> (w187:T17)  [unwired: 1 out]
        n129 = Initialize Array(0, w189) -> (w191:i32[])
        n130 = for {
          tunnel: w191 -> [w227] mode=indexing
          tunnel: [w225] -> w190 mode=indexing
          i -> [w226]
          n131 = Add(x=w227, y=w226) -> (x+y=w225:i32)
        }
        n132 = call "LC1_MS_Main.vi"("MS_Network_Settings"=w187, "Analog Output"=w215, "Analog Input Indexes"=w190) -> ("MS_DNP3_Settings"=w222:T7, "MS_RESET"=w221:bool, "Digital Input"=w218:bool[], "MS_ENABLE"=w220:bool, 10:w217, "Poll Enable"=w219:T9, 12:w185, "DNP3 Session Feedback"=w186:T16)  [unwired: 2 in, 3 out]
        n133 = Unbundle By Name(w186) -> ("error out"=→"error out")
      }
    }
    frame Enabled {
    }
  }
  n134 = disable-structure shown="Disabled" {
    frame Disabled {
      n135 = while {
        i -> [w236]
        stop <- w237 stop-if-true
        n136 = disable-structure shown="Disabled" {
          disable-tunnel: w236 -> [w238 _]
          frame Disabled {
            n137 = flat-sequence {
              tunnel: w238 -> [w254]
              frame #0 {
                n138 = case shown="True" {
                  selector: _ -> [_ _]
                  frame False {
                    n139 = global read "Global communication output.vi" "BESS Control"() -> (w239)
                    n140 = disable-structure shown="Disabled" {
                      disable-tunnel: w239 -> [w240 _]
                      frame Disabled {
                        n141 = shared-variable "LC1\\Variables for HTB.lvlib\\MGCC_to_BESS"(w240) -> ()  [unwired: 1 in, 1 out]
                      }
                      frame Enabled {
                      }
                    }
                  }
                  frame True {
                    n142 = case shown="False" w241 {
                      frame False {
                        n143 = global read "Global communication output.vi" "BESS Control"() -> (w242)
                        n144 = Replace Array Subset(array=w242, new element=0.0 ("new element/subarray"), index=0) -> (w243:dbl[])
                        n145 = disable-structure shown="Disabled" {
                          disable-tunnel: w243 -> [w246 _]
                          frame Disabled {
                            n146 = shared-variable "LC1\\Variables for HTB.lvlib\\MGCC_to_BESS"(w246) -> ()  [unwired: 1 in, 1 out]
                          }
                          frame Enabled {
                          }
                        }
                        n147 = global write "Global communication output.vi" "BESS Control"(w243) -> ()
                      }
                      frame True {
                        n148 = global read "Global communication output.vi" "BESS Control"() -> (w247)
                        n149 = Replace Array Subset(array=w247, new element=1.0 ("new element/subarray"), index=0) -> (w248:dbl[])
                        n150 = disable-structure shown="Disabled" {
                          disable-tunnel: w248 -> [w251 _]
                          frame Disabled {
                            n151 = shared-variable "LC1\\Variables for HTB.lvlib\\MGCC_to_BESS"(w251) -> ()  [unwired: 1 in, 1 out]
                          }
                          frame Enabled {
                          }
                        }
                        n152 = global write "Global communication output.vi" "BESS Control"(w248) -> ()
                      }
                    }
                  }
                }
              }
              frame #1 {
                n153 = disable-structure shown="Disabled" {
                  frame Disabled {
                    n154 = shared-variable "LC1\\Variables for HTB.lvlib\\BESS_to_MGCC"() -> (w252:dbl[])  [unwired: 1 in, 1 out]
                    n155 = global write "Global communication.vi" "BESS LC communication"(w252) -> ()
                  }
                  frame Enabled {
                  }
                }
              }
              frame #2 {
                n156 = Quotient & Remainder(x=w254, y=10) -> (x-y*floor(x/y)=w253:i32)  [unwired: 1 out]
              }
            }
            n157 = flat-sequence {
              tunnel: w238 -> [w270]
              frame #0 {
                n158 = disable-structure shown="Disabled" {
                  frame Disabled {
                  }
                  frame Enabled {
                  }
                }
                n159 = disable-structure shown="Disabled" {
                  frame Disabled {
                    n160 = global read "Global communication output.vi" "PV Control"() -> (w267:dbl[])
                  }
                  frame Enabled {
                  }
                }
                n161 = case shown="False" {
                  selector: _ -> [_ _]
                  frame False {
                    n162 = disable-structure shown="Disabled" {
                      frame Disabled {
                        n163 = global read "Global communication output.vi" "PV Control"() -> (w256:dbl[])
                        n164 = shared-variable "LC2\\Variables for HTB.lvlib\\MGCC_to_PV"(w256) -> ()  [unwired: 1 in, 1 out]
                      }
                      frame Enabled {
                      }
                    }
                  }
                  frame True {
                    n165 = case shown="True" w257 {
                      frame False {
                        n166 = shared-variable "LC2\\Variables for HTB.lvlib\\MGCC_to_PV"() -> (w261:dbl[])  [unwired: 1 in, 1 out]
                        n167 = Replace Array Subset(array=w261, new element=0.0 ("new element/subarray"), index=0) -> (w258:dbl[])
                        n168 = shared-variable "LC2\\Variables for HTB.lvlib\\MGCC_to_PV"(w258) -> ()  [unwired: 1 in, 1 out]
                        n169 = global write "Global communication output.vi" "PV Control"(w258) -> ()
                      }
                      frame True {
                        n170 = shared-variable "LC2\\Variables for HTB.lvlib\\MGCC_to_PV"() -> (w265:dbl[])  [unwired: 1 in, 1 out]
                        n171 = Replace Array Subset(array=w265, new element=1.0 ("new element/subarray"), index=0) -> (w262:dbl[])
                        n172 = disable-structure shown="Disabled" {
                          disable-tunnel: w262 -> [w266 _]
                          frame Disabled {
                            n173 = shared-variable "LC2\\Variables for HTB.lvlib\\MGCC_to_PV"(w266) -> ()  [unwired: 1 in, 1 out]
                          }
                          frame Enabled {
                          }
                        }
                        n174 = global write "Global communication output.vi" "PV Control"(w262) -> ()
                      }
                    }
                  }
                }
              }
              frame #1 {
                n175 = disable-structure shown="Disabled" {
                  frame Disabled {
                    n176 = shared-variable "LC2\\Variables for HTB.lvlib\\PV_to_MGCC"() -> (w268:dbl[])  [unwired: 1 in, 1 out]
                    n177 = global write "Global communication.vi" "PV LC communication"(w268) -> ()
                  }
                  frame Enabled {
                  }
                }
              }
              frame #2 {
                n178 = Quotient & Remainder(x=w270, y=10) -> (x-y*floor(x/y)=w269:i32)  [unwired: 1 out]
              }
            }
          }
          frame Enabled {
          }
        }
        n179 = disable-structure shown="Disabled" {
          disable-tunnel: w236 -> [w272 _]
          frame Disabled {
            # "IntellRupter"
            n180 = flat-sequence {
              tunnel: w272 -> [w276]
              frame #0 {
              }
              frame #1 {
                n181 = shared-variable "Relay Control\\LC_Relay_data.lvlib\\ar_Relay_to_MGCC"() -> (w273:dbl[])  [unwired: 1 in, 1 out]
                n182 = global write "Global communication.vi" "Global communication"(w273) -> ()
              }
              frame #2 {
              }
              frame #3 {
                n183 = Quotient & Remainder(x=w276, y=10) -> (x-y*floor(x/y)=w274:i32)  [unwired: 1 out]
              }
            }
          }
          frame Enabled {
          }
        }
        n184 = shared-variable "MGCC\\MGCC_FntStaMach_Finte State Machine.lvlib\\b_MGCC_FntStaMach_All_Loop_Stop"() -> (w237:bool)  [unwired: 1 in, 1 out]
        n185 = Wait (ms)(milliseconds to wait=u32 100) -> ()  [unwired: 1 out]
      }
    }
    frame Enabled {
    }
  }
  n186 = disable-structure shown="Disabled" {
    frame Disabled {
      n187 = while {
        i -> [w320]
        stop <- FALSE stop-if-true
        (unwired) u16[] [0, 1, 2, 3, 4, 5, 6] ("Analog Input Indexes")
        n188 = global read "Global communication output.vi" "PV Control"() -> (w311:dbl[])
        n189 = global read "MGCC_Global_communication_inputsettings .vi" "DNP3 Outstation Address PV"() -> (w285:dbl)
        n190 = global read "MGCC_Global_communication_inputsettings .vi" "DNP3 Master Address PV"() -> (w286:dbl)
        n191 = global read "MGCC_Global_communication_inputsettings .vi" "DNP3 port PV"() -> (w287:dbl)
        n192 = global read "MGCC_Global_communication_inputsettings .vi" "IP_PV"() -> (w289:dbl[])
        n193 = for {
          tunnel: [w331] -> w312 mode=indexing
          tunnel: w311 -> [w326] mode=indexing
          i -> [w325]
          n194 = To Unsigned Word Integer(number=w325) -> (unsigned 16bit integer=w327:u16)
          n195 = Index Array(array=T1[] [] ("values"), index=0) -> (element=w328:T1)
          n196 = Bundle(cluster=w328, "index"=w327, "value"=w326) -> (w331:T1)
        }
        n197 = Number To Decimal String(number=w289, width (-)=i16 3) -> (decimal integer string=w306:string[])
        n198 = Index Array(array=w306, index #1=0 ("index"), index #2=1 ("index"), index #3=2 ("index"), index #4=3 ("index")) -> (element #1=w298:string, element #2=w296:string, element #3=w294:string, element #4=w292:string)
        n199 = call <vilib>:"Trim Whitespace.vi"("string"=w298) -> ("trimmed string"=w297:string)  [unwired: 1 in]
        n200 = call <vilib>:"Trim Whitespace.vi"("string"=w296) -> ("trimmed string"=w295:string)  [unwired: 1 in]
        n201 = call <vilib>:"Trim Whitespace.vi"("string"=w294) -> ("trimmed string"=w293:string)  [unwired: 1 in]
        n202 = call <vilib>:"Trim Whitespace.vi"("string"=w292) -> ("trimmed string"=w291:string)  [unwired: 1 in]
        n203 = feedback #3() -> (w315)  [unwired: 1 in]
        n204 = Concatenate Strings(w297, "." ("string"), w295, "." ("string"), w293, "." ("string"), w291) -> (w288:string)
        n205 = Bundle(w288, "DNP3 port PV"=w287, "DNP3 Master Address PV"=w286, "DNP3 Outstation Address PV"=w285) -> (w283:T18, w284:T18)
        n206 = global read "MGCC_Global_communication_inputsettings .vi" "Analogue control channel number PV"() -> (w282:dbl)
        n207 = Equal?(x=Response_Type."Success" ("LC1_MS_RX_Status_Analog 2")) -> (y=w308:T8, x = y?=w307:bool)
        n208 = Initialize Array(0, w282) -> (w280:i32[])
        n209 = shared-variable "MGCC\\MGCC_comm_lib.lvlib\\b_MGCC_Commun_enable"(w307) -> ()  [unwired: 1 in, 1 out]
        n210 = for {
          tunnel: w280 -> [w324] mode=indexing
          tunnel: [w322] -> w279 mode=indexing
          i -> [w323]
          n211 = Add(x=w324, y=w323) -> (x+y=w322:i32)
        }
        n212 = call "LC1_MS_Main.vi"("MS_Network_Settings"=w283, "Analog Output"=w312, "Analog Input Indexes"=w279, 12:w315) -> ("Comm Status"=→"MS SETTINGS CHANGED 2":T15, "MS_DNP3_Settings"=w319:T7, "MS_RESET"=w318:bool, "Digital Input"=w313:bool[], "MS_ENABLE"=w317:bool, 10:w310, "Poll Enable"=w316:T9, "DNP3 Session Feedback"=w277:T16)  [unwired: 2 in, 2 out]
        n213 = Unbundle By Name(w277) -> ("error out"=→"error out 2")
        n214 = feedback-in #3(w277) -> ()
        n215 = global write "Global communication.vi" "PV LC communication"(w310) -> ()
      }
    }
    frame Enabled {
    }
  }
  n216 = disable-structure shown="Disabled" {
    frame Disabled {
      n217 = while {
        shift-right: [w356] -> _
        shift-left: _ -> [w355]
        stop <- FALSE stop-if-true
        w342 = 1 ("y")
        n218 = local read "error out 2"() -> (w352:errorcluster)
        n219 = local read "error out"() -> (w353:errorcluster)
        n220 = local read "error out 3"() -> (w332:errorcluster)
        n221 = Wait (ms)(milliseconds to wait=u32 2000) -> ()  [unwired: 1 out]
        n222 = local read item#-1() -> (w338)
        n223 = local read "Numeric"() -> (w336:i32)
        n224 = Unbundle By Name(w353) -> ("code"=w350:i32)
        n225 = Unbundle By Name(w352) -> ("code"=w351:i32)
        n226 = feedback #4() -> (w337:i32)  [unwired: 1 in]
        n227 = feedback-in #4(w336) -> ()
        n228 = feedback #5() -> (w339)  [unwired: 1 in]
        n229 = feedback-in #5(w338) -> ()
        n230 = Unbundle By Name(w332) -> ("code"=w354:i32)
        n231 = Subtract(x=w336, y=w337) -> (x-y=w340:i32)
        n232 = Subtract(x=w338, y=w339) -> (x-y=w341:dbl)
        n233 = Not Equal To 0?(x=w350) -> (x != 0?=w348:bool)
        n234 = Not Equal To 0?(x=w351) -> (x != 0?=w347:bool)
        n235 = Not Equal To 0?(x=w354) -> (x != 0?=w349:bool)
        n236 = Less?(x=w341, y=w342) -> (x < y?=w344:bool)
        n237 = Less?(x=w340, y=w342) -> (x < y?=w343:bool)
        n238 = Compound Arithmetic op=OR(w349, w348, w347) -> (w346:bool)
        n239 = xnode "Error Ring"() -> ("error out"=w335:errorcluster)
        n240 = case shown="True" w346 {
          tunnel: [0 w370] -> w356
          tunnel: w355 -> [_ w376]
          frame False {
            n241 = xnode "Error Ring"() -> ("error out"=w365:errorcluster)
            n242 = shared-variable "MGCC\\MGCC_comm_lib.lvlib\\e_MGCC_Commun_error"(w365) -> ()  [unwired: 1 in, 1 out]
          }
          frame True {
            w371 = 150 ("y")
            w369 = 30 ("y")
            n243 = Increment(x=w376) -> (x+1=w370:i32)
            n244 = Greater?(x=w371, y=w370) -> (0:w373:bool)
            n245 = Greater Or Equal?(x=w370, y=w371) -> (x >= y?=w375:bool)
            n246 = Greater Or Equal?(x=w370, y=w369) -> (x >= y?=w374:bool)
            n247 = And(x=w373, y=w374) -> (x .and. y?=w372:bool)
            n248 = Greater?(x=w369, y=w370) -> (0:w368:bool)
            n249 = case shown="True" w372 {
              frame False {
              }
              frame True {
                n250 = xnode "Error Ring"() -> ("error out"=w387:errorcluster)
                n251 = shared-variable "MGCC\\MGCC_comm_lib.lvlib\\e_MGCC_Commun_error"(w387) -> ()  [unwired: 1 in, 1 out]
              }
            }
            n252 = case shown="True" w375 {
              frame False {
              }
              frame True {
                n253 = xnode "Error Ring"() -> ("error out"=w381:errorcluster)
                n254 = shared-variable "MGCC\\MGCC_comm_lib.lvlib\\e_MGCC_Commun_error"(w381) -> ()  [unwired: 1 in, 1 out]
              }
            }
            n255 = case shown="True" w368 {
              frame False {
              }
              frame True {
                n256 = local read "error out 3"() -> (w380:errorcluster)
                n257 = local read "error out"() -> (w379:errorcluster)
                n258 = local read "error out 2"() -> (w378:errorcluster)
                n259 = Merge Errors(w380, w379, w378) -> (w377:errorcluster)
                n260 = shared-variable "MGCC\\MGCC_comm_lib.lvlib\\e_MGCC_Commun_error"(w377) -> ()  [unwired: 1 in, 1 out]
              }
            }
          }
        }
        n261 = xnode "Error Ring"() -> ("error out"=w334:errorcluster)
        n262 = Or(x=w343, y=w344) -> (x .or. y?=w333:bool)
        n263 = Select(t=w335, s=w333, f=w334) -> (s? t:f=→"error out 3":errorcluster)
      }
    }
    frame Enabled {
    }
  }
